vi "Front_to_access_test1.vi"(8 "error in (no error) 2":errorcluster) -> (0 "error in (no error)":errorcluster)   [LabVIEW 2017]
uses:
  b5ca2ae4-87b0-45ed-966a-308aef782838.vi
  af378c36-64ad-42fa-a7d2-44d916e06ec5.vi
panel:
  in  "String":string
  # "Thi is auto vi"
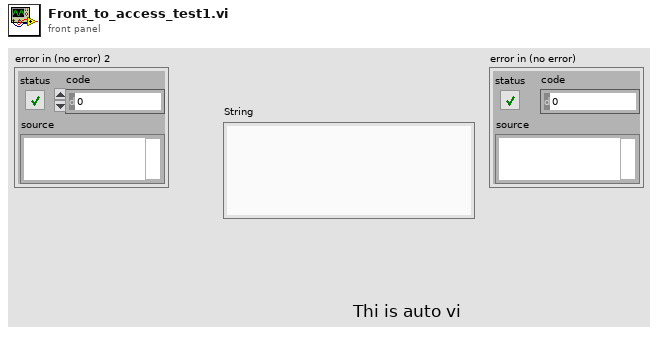
[diagram p1: front panel]
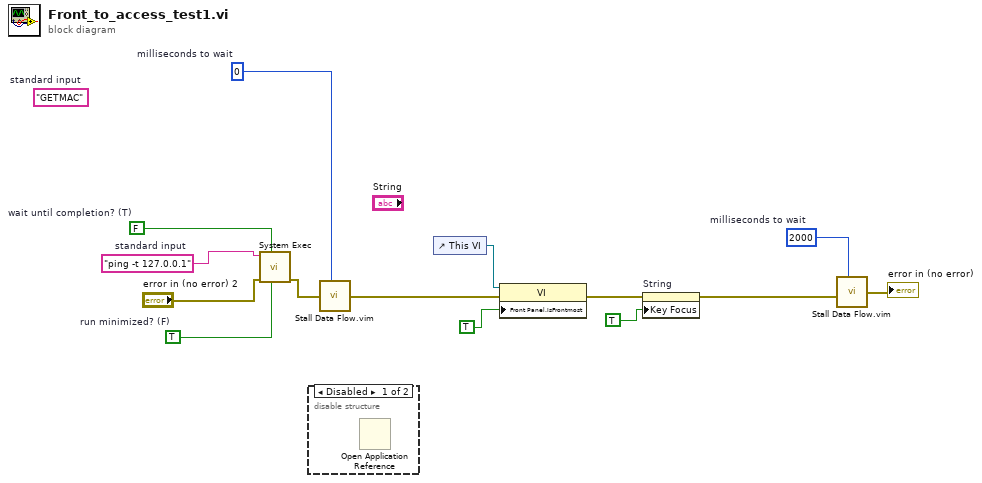
[diagram p0: block diagram]
diagram:
  w2 = FALSE  # wait until completion? (T)
  (unwired) "GETMAC"  # standard input
  w5 = u32 2000  # milliseconds to wait
  w8 = TRUE  # run minimized? (F)
  w1 = "ping -t 127.0.0.1"  # standard input
  w14 = u32 0  # milliseconds to wait
  n1 = call <vilib>:"System Exec.vi"("run minimized? (F)"=w8, "wait until completion? (T)"=w2, "error in (no error)"="error in (no error) 2", "command line"=w1) -> ("error out"=w9:errorcluster)  [unwired: 4 in, 3 out]
  n2 = disable-structure shown="Disabled" {
    frame Disabled {
      n3 = Open Application Reference() -> ()  [unwired: 4 in, 2 out]
    }
    frame Enabled {
    }
  }
  n4 = call "Stall Data Flow.vim"("value in"=w9, "milliseconds to wait"=w14) -> ("value out"=w13:errorcluster)  [unwired: 1 out]
  n5 = control-ref of="This VI"() -> (w4:refnum<vi>)
  n6 = property class="VI"(reference=w4, error in=w13, "Front Panel.IsFrontmost"=TRUE) -> (error out=w11:errorcluster)  [unwired: 1 out]
  n7 = property on="String" class="Str"(error in=w11, "Key Focus"=TRUE) -> (error out=w7:errorcluster)  [unwired: 1 in, 1 out]
  n8 = call "Stall Data Flow.vim"("value in"=w7, "milliseconds to wait"=w5) -> ("value out"=→"error in (no error)":errorcluster)  [unwired: 1 out]
